vi "portUtil.vi"(5 "Register":u8, 7 "Destination":u8, 8 "error in (no error)":errorcluster, 9 "WriteNotRead":bool, 10 "Array":u8[](array[numeric]), 11 "COMport":string="COM6") -> (0 "error out":errorcluster, 1 "PayloadByteArray":u8[](array[numeric]), 2 "Long":i32)   [LabVIEW 2015]
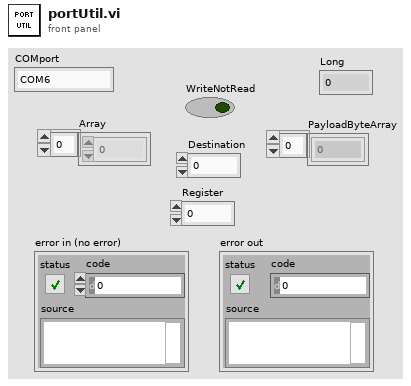
[diagram p1: front panel]
types:
  T1 = cluster{"Destination":u8, "Source":u8, "Register":u8, "Array":i16[], "WriteNotRead":bool, "ReadWithPreample":bool, "Ring":u16, "String":string, "Long":i32}
  T2 = cluster{"OpenPort":bool, "ClosePort":bool, "Baudrate":i32, "Wait":u16, "ReadWrite":bool}
  T3 = cluster{"Source":u8, "TelegramType":u8, "Register":u8, "Destination":u8, "TelegramReceived":bool, "CRC error":bool, "PayloadByteArray":u8[], "(hi.lo)":u16, "Crc16":u16, "Long":i32, "PayloadIntArray":u16[], "String":string}
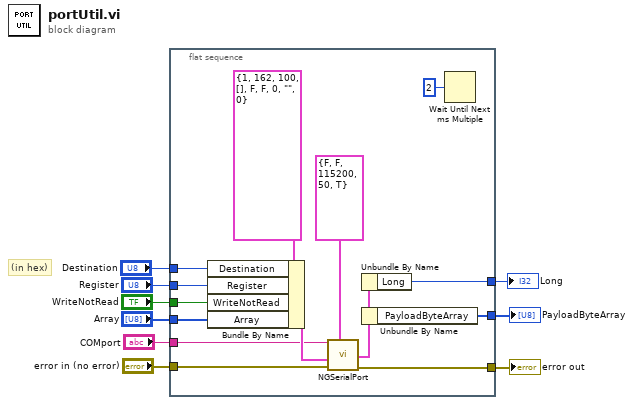
[diagram p0: block diagram]
diagram:
  # "(in hex)"
  n1 = flat-sequence {
    tunnel: "WriteNotRead" -> [w21]
    tunnel: "Destination" -> [w19]
    tunnel: "Register" -> [w18]
    tunnel: [w17] -> w6
    tunnel: "error in (no error)" -> [w16]
    tunnel: "COMport" -> [w15]
    tunnel: "Array" -> [w13]
    tunnel: [w12] -> w3
    tunnel: [w10] -> w2
    frame #0 {
      n2 = Bundle By Name(cluster=T1 {"Destination"=1, "Source"=162, "Register"=100, "Array"=[], "WriteNotRead"=FALSE, "ReadWithPreample"=FALSE, "Ring"=0, "String"="", "Long"=0} ("InParameters"), "Destination"=w19, "Register"=w18, "WriteNotRead"=w21, "Array"=w13) -> (w20:T1)
      n3 = call "NGSerialPort.vi"("PortParameters"=T2 {"OpenPort"=FALSE, "ClosePort"=FALSE, "Baudrate"=115200, "Wait"=50, "ReadWrite"=TRUE}, "error in"=w16, "InParameters"=w20, "VISA in"=w15) -> ("error out"=w17:errorcluster, "OutParameters"=w11:T3)  [unwired: 5 in, 1 out]
      n4 = Unbundle By Name(w11) -> ("Long"=w10:i32)
      n5 = Unbundle By Name(w11) -> ("PayloadByteArray"=w12:u8[])
      n6 = Wait Until Next ms Multiple(millisecond multiple=u32 2) -> ()  [unwired: 1 out]
    }
  }
  "error out" <- w6
  "PayloadByteArray" <- w3
  "Long" <- w2
